vi "HMP231.vi"(4 "Channel Name":string, 5 "Port Name":string, 6 "Channel":T1(ring), 7 "Address":u8=50) -> (0 "Output":dbl format="%.2f", 3 "Status note":string)   [LabVIEW 2010]
panel:
  out "Numerics":dbl[](array[numeric])=[nan, nan, nan] format="%.2f"
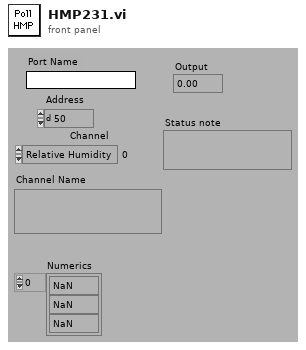
[diagram p1: front panel]
types:
  T1 = enum16{"Relative Humidity", "Temperature", "Dewpoint"}
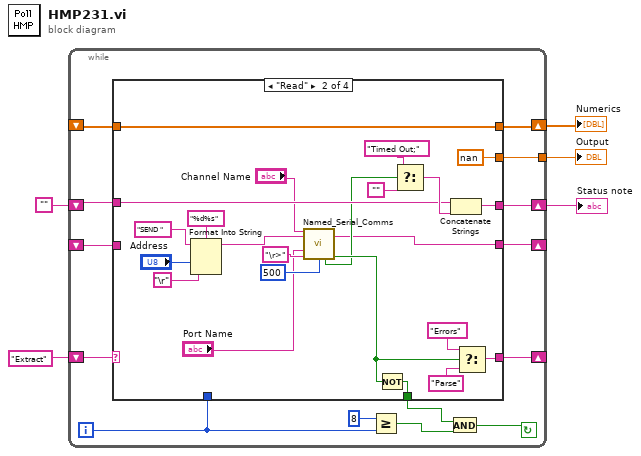
[diagram p0: block diagram]
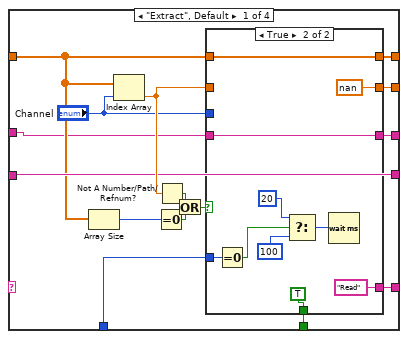
[diagram p2: hidden frame]
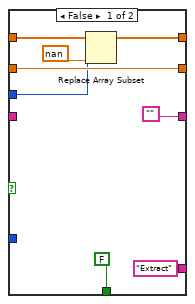
[diagram p3: hidden frame]
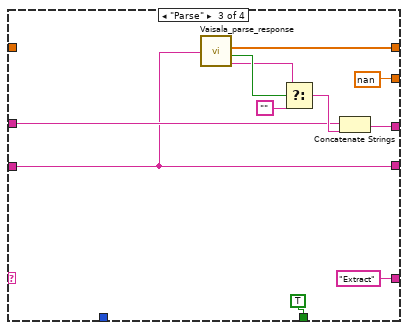
[diagram p4: hidden frame]
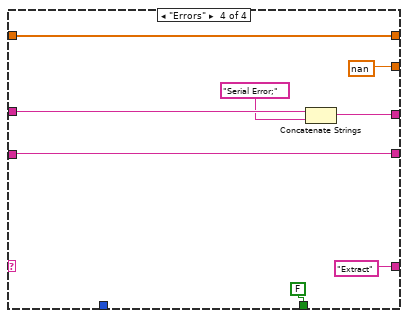
[diagram p5: hidden frame]
diagram:
  n1 = while {
    shift-left: _ -> [w11]
    shift-right: [w12] -> _
    shift-left: "" -> [w13]
    shift-right: [w14] -> w3
    shift-left: "Extract" -> [w16]
    shift-right: [w15] -> _
    tunnel: [w17] -> w5
    shift-left: _ -> [w18]
    shift-right: [w19] -> w1
    i -> [w6]
    stop <- w7 continue-if-true
    n2 = case shown="\"Read\"" w16 {
      tunnel: [w29 w75 w86 w92] -> w19
      tunnel: w18 -> [w27 w75 _ w92]
      tunnel: [w33 nan nan nan] -> w17
      tunnel: [w31 w68 "Extract" "Extract"] -> w15
      tunnel: [w32 w65 TRUE FALSE] -> w8
      tunnel: [w22 w61 w82 w90] -> w14
      tunnel: w13 -> [w21 w60 w81 w89]
      tunnel: [w28 w58 w76 w87] -> w12
      tunnel: w11 -> [w28 _ w76 w87]
      tunnel: w6 -> [w20 _ _ _]
      frame "Extract", Default {
        n3 = Array Size(array=w27) -> (size(s)=w26:i32)
        n4 = Index Array(array=w27, index="Channel") -> (element=w34:dbl)
        n5 = Equal To 0?(x=w26) -> (x = 0?=w24:bool)
        n6 = Not A Number/Path/Refnum?(number/path/refnum=w34) -> (NaN/Path/Refnum?=w25:bool)
        n7 = Or(x=w25, y=w24) -> (x .or. y?=w23:bool)
        n8 = case shown="True" w23 {
          tunnel: w34 -> [w42 _]
          tunnel: [w42 nan] -> w33
          tunnel: [FALSE TRUE] -> w32
          tunnel: ["Extract" "Read"] -> w31
          tunnel: w27 -> [w39 w52]
          tunnel: "Channel" -> [w37 _]
          tunnel: [w36 w52] -> w29
          tunnel: ["" w48] -> w22
          tunnel: w21 -> [_ w48]
          tunnel: w20 -> [_ w47]
          frame False {
            n9 = Replace Array Subset(array=w39, new element=nan, index=w37) -> (w36:dbl[])
          }
          frame True {
            n10 = Equal To 0?(x=w47) -> (x = 0?=w46:bool)
            n11 = Select(t=u32 20, s=w46, f=u32 100 ("milliseconds to wait")) -> (s? t:f=w45:u32)
            n12 = Wait (ms)(milliseconds to wait=w45) -> ()  [unwired: 1 out]
          }
        }
      }
      frame "Read" {
        n13 = Format Into String(format string="%d%s" ("Format String"), initial string="SEND " ("Input String"), "Address", "\r") -> (resulting string=w74:string)  [unwired: 1 in, 1 out]
        n14 = call "Named_Serial_Comms.vi"("Channel Name"="Channel Name", "Write String"=w74, "Timeout/ms"=u32 500 ("Timeout"), "Port Name"="Port Name", "Term Grep"="\r>") -> ("Read"=w58:string, "Timed out"=w59:bool, "Serial Error"=w66:bool)  [unwired: 4 in, 4 out]
        n15 = Not(x=w66) -> (.not. x?=w65:bool)
        n16 = Select(t="Timed Out;", s=w59, f="") -> (s? t:f=w63:string)
        n17 = Concatenate Strings(w60, w63) -> (w61:string)
        n18 = Select(t="Errors", s=w66, f="Parse") -> (s? t:f=w68:string)
      }
      frame "Parse" {
        n19 = call "Vaisala_parse_response.vi"("HMP response string"=w76) -> ("Numerics"=w86:dbl[], "Error"=w80:bool, "Error notes"=w79:string)  [unwired: 3 out]
        n20 = Select(t=w79, s=w80, f="") -> (s? t:f=w84:string)
        n21 = Concatenate Strings(w81, w84) -> (w82:string)
      }
      frame "Errors" {
        n22 = Concatenate Strings(w89, "Serial Error;" ("t")) -> (w90:string)
      }
    }
    n23 = Greater Or Equal?(x=8, y=w6) -> (x >= y?=w9:bool)
    n24 = And(x=w8, y=w9) -> (x .and. y?=w7:bool)
  }
  "Status note" <- w3
  "Output" <- w5
  "Numerics" <- w1
